vi "Exit.vi"(8 "error in":errorcluster, 11 "SignalWriterMH110203USBStepperMotor.lvclass":refnum<class "SignalWriterMH110203USBStepperMotor.lvclass">) -> (0 "error out":errorcluster, 3 "SignalWriterMH110203USBStepperMotor.lvclass 2":refnum<class "SignalWriterMH110203USBStepperMotor.lvclass">)   [LabVIEW 2010, in "SignalWriterMH110203USBStepperMotor.lvclass"]
uses:
  SignalWriterMH110203USBStepperMotor.lvclass
  SignalWriterMH110203USBStepperMotor.lvclass/SignalWriterMH110203USBStepperMotor.ctl
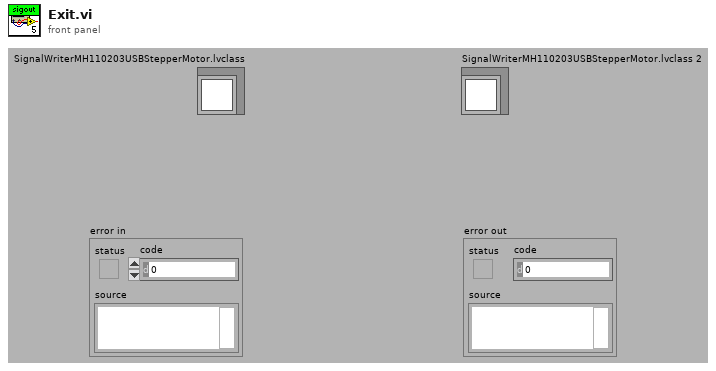
[diagram p1: front panel]
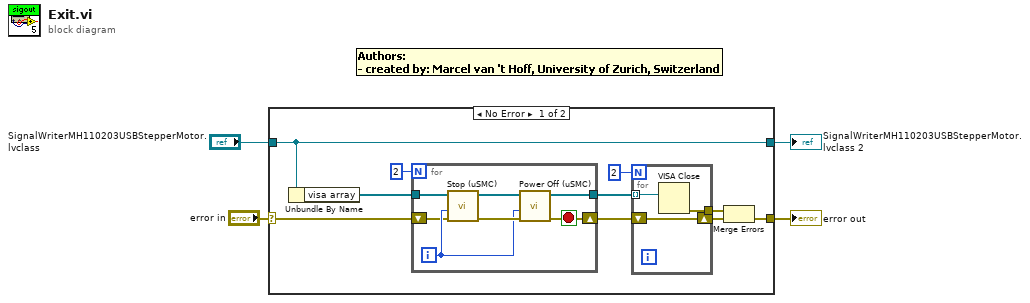
[diagram p0: block diagram]
diagram:
  n1 = case shown="No Error" "error in" {
    selector: "error in" -> [w14 w26]
    tunnel: [w5 w26] -> w4
    tunnel: "SignalWriterMH110203USBStepperMotor.lvclass" -> [w12 w25]
    tunnel: [w12 w25] -> w1
    frame No Error {
      n2 = Unbundle By Name(w12) -> ("visa array"=w13:refnum<visa-resource-name>[])
      n3 = for {
        N: 2 -> [_]
        tunnel: w13 -> [w23]
        tunnel: [w18] -> w11
        shift-right: [w19] -> w8
        shift-left: w14 -> [w20]
        i -> [w21]
        stop <- w19 stop-if-true
        n4 = call "Stop (uSMC).vi"("error in (no error)"=w20, "Index"=w21, "Visa array in"=w23) -> ("error out"=w24:errorcluster, "Visa array out"=w22:refnum<visa-resource-name>[])  [unwired: 7 in]
        n5 = call "Power Off (uSMC).vi"("error in (no error)"=w24, "Index"=w21, "Visa Array in"=w22) -> ("error out"=w19:errorcluster, "Visa Array out"=w18:refnum<visa-resource-name>[])  [unwired: 7 in]
      }
      n6 = for {
        N: 2 -> [_]
        tunnel: w11 -> [w17] mode=indexing
        tunnel: [w15] -> w7
        shift-right: [w16] -> w6
        shift-left: w8 -> [w16]
        n7 = VISA Close(VISA resource name=w17) -> (error out=w15:errorcluster)  [unwired: 1 in]
      }
      n8 = Merge Errors(w7, w6) -> (w5:errorcluster)
    }
    frame Error {
    }
  }
  "error out" <- w4
  "SignalWriterMH110203USBStepperMotor.lvclass 2" <- w1
